vi "integrate position.vi"() -> ()   [LabVIEW 2009]
panel:
  in  "parameters":T1={"max velocity (m/s)"=2.0, "wheel base width (m)"=0.7, "traverse CoF"=0.14}
  out "Array":dbl[](array[numeric])
  out "XY Graph":cluster{dbl, dbl}[](graph)
  in  "iterations":i32=120
  in  "Ætime (s)":dbl=0.01
  in  "initial m/s":dbl(slide)=1.5918367346938773 scale=-2.0..2.0
  in  "initial direction":dbl(knob) scale=6.28..0.0
  in  "% turn":dbl(slide)=100.0 scale=-100.0..100.0
  in  "m/s/s":dbl(slide)=0.693877551020408 scale=-1.0..1.0
  # "Integrate position:\niteratively run \"calcuclate position\", incrementing along"
  # "PROBLEM:\nsharp turn at speed 1.7 and 2.0"
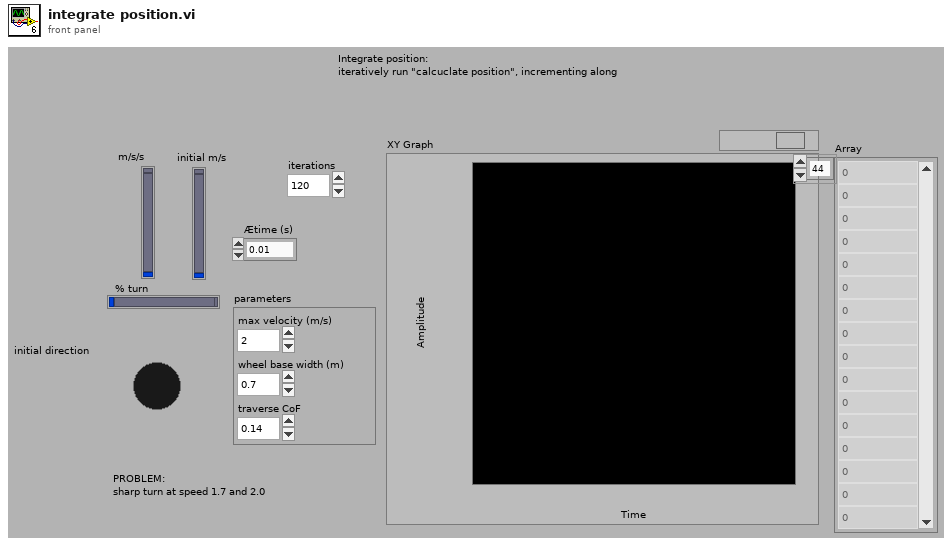
[diagram p1: front panel]
types:
  T1 = cluster{"max velocity (m/s)":dbl, "wheel base width (m)":dbl, "traverse CoF":dbl}
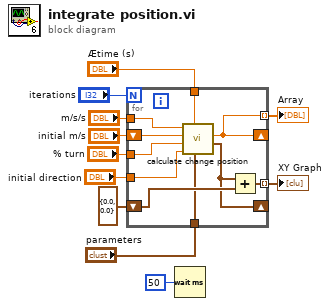
[diagram p0: block diagram]
diagram:
  n1 = for {
    N: "iterations" -> [_]
    shift-right: [w13] -> _
    shift-left: "initial m/s" -> [w21]
    tunnel: "m/s/s" -> [w20]
    tunnel: "% turn" -> [w19]
    tunnel: "initial direction" -> [w18]
    shift-right: [w15] -> _
    shift-left: cluster{dbl, dbl} {0.0, 0.0} ("Æ point") -> [w16]
    tunnel: "Ætime (s)" -> [w17]
    tunnel: [w14] -> w4 mode=indexing
    tunnel: [w13] -> w3 mode=indexing
    tunnel: "parameters" -> [w12]
    n2 = call "calculate change position.vi"("parameters"=w12, "Ætime (s)"=w17, "initial direction"=w18, "% turn"=w19, "m/s"=w21, "m/s/s"=w20) -> ("Æ point"=w15:cluster{dbl, dbl}, "end velocity (m/s)"=w13:dbl)  [unwired: 4 in]
    n3 = Add(x=w15, y=w16) -> (x+y=w14:cluster{dbl, dbl})
  }
  "XY Graph" <- w4
  "Array" <- w3
  n4 = Wait (ms)(milliseconds to wait=u32 50) -> ()  [unwired: 1 out]
